vi "Serial Communcation Devices Initialization VI.vi"(8 "error in (no error)":errorcluster, 10 "Custom XML":string, 11 "Device Item Ref in":T1) -> (0 "error out":errorcluster, 3 "Device Item Ref out":T1 format="%.0x")   [LabVIEW 2017, in "Serial Communcation Devices Custom Device.lvlib"]
uses:
  Serial Communcation Devices Custom Device.lvlib
  <vilib>/NI Veristand/Custom Device API/Custom Device Item Ref.ctl
  <vilib>/NI Veristand/Custom Device API/Custom Device Channel Type.ctl
  <vilib>/NI Veristand/Custom Device API/Set Item Property (Boolean).vi
  <vilib>/NI Veristand/Custom Device API/Set Item Property (U16).vi
  <vilib>/NI Veristand/Custom Device API/Set Item Property (String).vi
  <vilib>/NI Veristand/Custom Device API/Custom Device API.lvlib
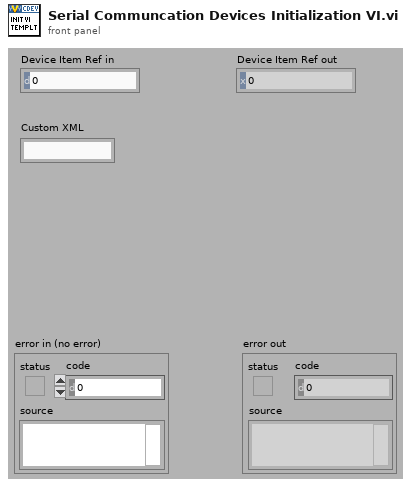
[diagram p1: front panel]
types:
  T1 = typedef "Custom Device API.lvlib/Custom Device Item Ref.ctl" = u64
  T2 = typedef "Custom Device API.lvlib/Custom Device Channel Type.ctl" = enum16{"Input", "Output"}
  T3 = cluster{"Type":T2, "Units":string, "Default Value":dbl, "Faultable":bool, "Scalable":bool}
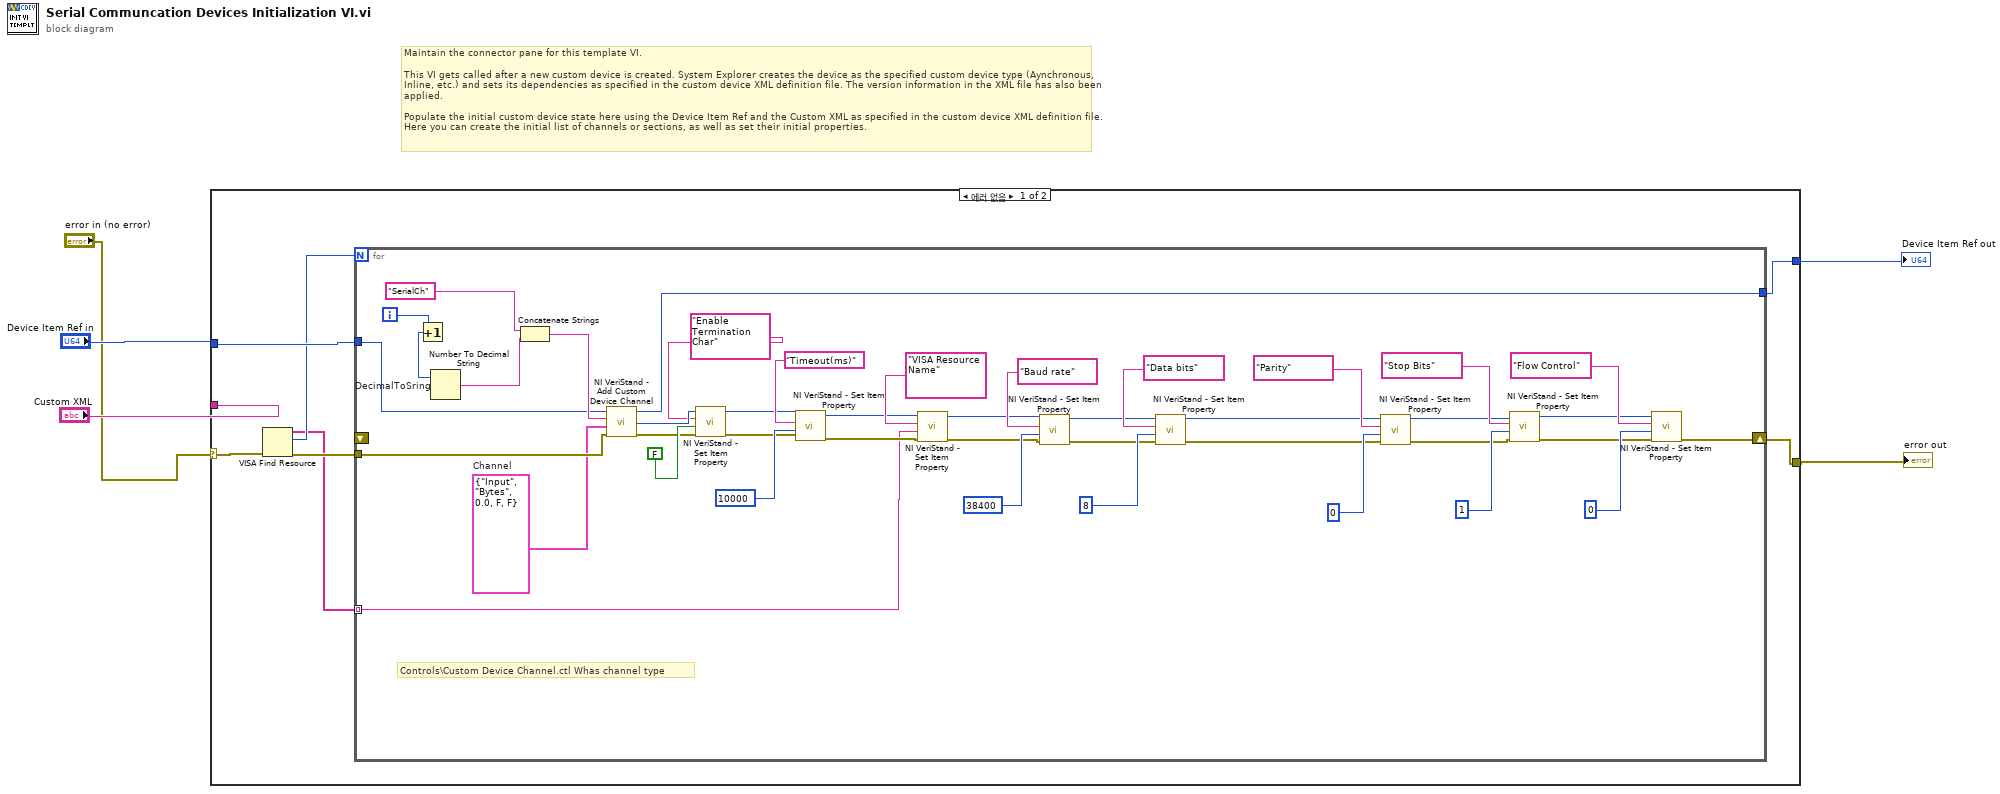
[diagram p0: block diagram]
diagram:
  # "Maintain the connector pane for this template VI.\n\nThis VI gets called after a new custom device is created. System Explorer creates the device as the specified custom device type (Aynchronous, Inline, etc.) and sets its dependencies as specified in the custom device XML definition file. The version information in the XML file has also been applied.\n\nPopulate the initial custom device state here using the Device Item Ref and the Custom XML as specified in the custom device XML definition file. Here you can create the initial list of channels or sections, as well as set their initial properties."
  n1 = case shown="에러 없음" "error in (no error)" {
    selector: "error in (no error)" -> [w8 w56]
    tunnel: [w11 w56] -> w3
    tunnel: [w10 w55] -> w2
    tunnel: "Device Item Ref in" -> [w12 w55]
    tunnel: "Custom XML" -> [_ _]
    frame No Error {
      n2 = VISA Find Resource(8:w8) -> (0:w7:errorcluster, 2:w9:u32, 3:w6:string[])  [unwired: 2 in]
      n3 = for {
        N: w9 -> [_]
        tunnel: w7 -> [w25]
        tunnel: w12 -> [w22]
        tunnel: [w16] -> w10
        shift-right: [w17] -> w11
        shift-left: _ -> [_]
        tunnel: w6 -> [w14] mode=indexing
        i -> [w24]
        w18 = T3 {"Type"=enum."Input", "Units"="Bytes", "Default Value"=0.0, "Faultable"=FALSE, "Scalable"=FALSE}  # Channel
        # "Controls\\Custom Device Channel.ctl Whas channel type"
        n4 = Increment(x=w24) -> (x+1=w19:i32)
        n5 = Number To Decimal String "DecimalToSring"(number=w19) -> (decimal integer string=w20:string)  [unwired: 1 in]
        n6 = Concatenate Strings("SerialCh", w20) -> (w23:string)
        n7 = call <vilib>:"NI VeriStand - Add Custom Device Channel.vi"("error in (no error)"=w25, "Channel"=w18, "Channel Name"=w23, "Parent Ref in"=w22) -> ("error out"=w37:errorcluster, "Channel Ref"=w15:T1, "Parent Ref out"=w16:T1)  [unwired: 4 in, 1 out]
        n8 = call-poly <vilib>:"NI VeriStand - Set Item Property.vi"("error in (no error)"=w37, "Value"=FALSE, "Property Name"="Enable Termination Char", "Item Ref in"=w15) -> ("error out"=w36:errorcluster, "Item Ref out"=w29:T1)  [unwired: 5 in, 1 out]
        n9 = call-poly <vilib>:"NI VeriStand - Set Item Property.vi"("error in (no error)"=w36, "Value"=10000, "Property Name"="Timeout(ms)", "Item Ref in"=w29) -> ("error out"=w35:errorcluster, "Item Ref out"=w28:T1)  [unwired: 5 in, 1 out]
        n10 = call-poly <vilib>:"NI VeriStand - Set Item Property.vi"("error in (no error)"=w35, "Value"=w14, "Property Name"="VISA Resource Name", "Item Ref in"=w28) -> ("error out"=w34:errorcluster, "Item Ref out"=w27:T1)  [unwired: 5 in, 1 out]
        n11 = call-poly <vilib>:"NI VeriStand - Set Item Property.vi"("error in (no error)"=w34, "Value"=38400, "Property Name"="Baud rate", "Item Ref in"=w27) -> ("error out"=w33:errorcluster, "Item Ref out"=w26:T1)  [unwired: 5 in, 1 out]
        n12 = call-poly <vilib>:"NI VeriStand - Set Item Property.vi"("error in (no error)"=w33, "Value"=8, "Property Name"="Data bits", "Item Ref in"=w26) -> ("error out"=w32:errorcluster, "Item Ref out"=w40:T1)  [unwired: 5 in, 1 out]
        n13 = call-poly <vilib>:"NI VeriStand - Set Item Property.vi"("error in (no error)"=w32, "Value"=0, "Property Name"="Parity", "Item Ref in"=w40) -> ("error out"=w31:errorcluster, "Item Ref out"=w39:T1)  [unwired: 5 in, 1 out]
        n14 = call-poly <vilib>:"NI VeriStand - Set Item Property.vi"("error in (no error)"=w31, "Value"=1, "Property Name"="Stop Bits", "Item Ref in"=w39) -> ("error out"=w30:errorcluster, "Item Ref out"=w38:T1)  [unwired: 5 in, 1 out]
        n15 = call-poly <vilib>:"NI VeriStand - Set Item Property.vi"("error in (no error)"=w30, "Value"=0, "Property Name"="Flow Control", "Item Ref in"=w38) -> ("error out"=w17:errorcluster)  [unwired: 5 in, 2 out]
      }
    }
    frame Error {
    }
  }
  "error out" <- w3
  "Device Item Ref out" <- w2
